vi "Messaging AE.vi"(5 "VI Refnum":refnum<vi>, 7 "Action":T1=enum."Get", 8 "Error In":errorcluster) -> (0 "Error Out":errorcluster, 3 "queue out":refnum<queue>)   [LabVIEW 2019, in "GUI.lvlib"]
doc: "<b>Action</b> Engine\nCreate: Obtains a Queue named after the VI.\nGet: Returns the Queue reference.\nDestroy: Releases the Queue.\n\nUse this VI before and after the main loop. Use the Get action in new APIs."
uses:
  GUI.lvlib
  Controls/Messaging Actions.ctl
  Controls/Messaging Data.ctl
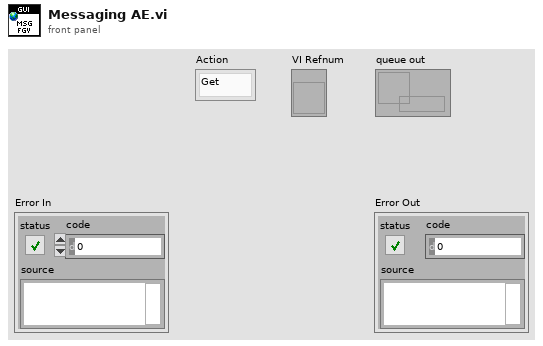
[diagram p1: front panel]
types:
  T1 = typedef "GUI.lvlib/Messaging Actions.ctl" = enum16{"Create", "Get", "Destroy"}
  T2 = typedef "GUI.lvlib/Messaging Data.ctl" = cluster{"Command":string, "Data":variant}
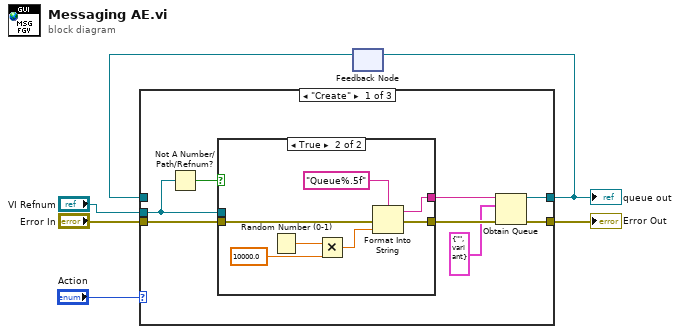
[diagram p0: block diagram]
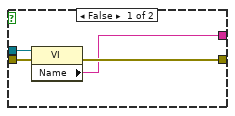
[diagram p2: hidden frame]
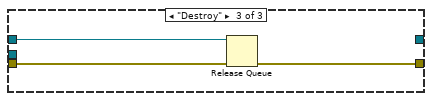
[diagram p4: hidden frame]
diagram:
  n1 = feedback #1() -> (w4:refnum<queue>)  [unwired: 1 in]
  n2 = case shown="\"Create\"" "Action" {
    tunnel: "Error In" -> [w14 w26 w30]
    tunnel: [w7 w26 w29] -> w5
    tunnel: [w12 w27 _] -> w3
    tunnel: w4 -> [_ w27 w28]
    tunnel: "VI Refnum" -> [w11 _ _]
    frame "Create" {
      n3 = Not A Number/Path/Refnum?(number/path/refnum=w11) -> (NaN/Path/Refnum?=w10:bool)
      n4 = case shown="True" w10 {
        tunnel: w14 -> [w18 w25]
        tunnel: [w17 w22] -> w13
        tunnel: w11 -> [w16 _]
        tunnel: [w15 w19] -> w9
        frame False {
          n5 = property class="VI"(reference=w16, error in=w18) -> (error out=w17:errorcluster, "Name"=w15:string)  [unwired: 1 out]
        }
        frame True {
          n6 = Random Number (0-1)() -> (number: 0 to 1=w24:dbl)
          n7 = Multiply(x=w24, y=10000.0) -> (x*y=w21:dbl)
          n8 = Format Into String(format string="Queue%.5f", error in=w25, w21) -> (resulting string=w19:string, error out=w22:errorcluster)  [unwired: 1 in]
        }
      }
      n9 = Obtain Queue(name (unnamed)=w9, element data type=T2 {"Command"="", "Data"=variant} ("Message Data"), error in (no error)=w13) -> (queue out=w12:refnum<queue>, error out=w7:errorcluster)  [unwired: 2 in, 1 out]
    }
    frame "Get", Default {
    }
    frame "Destroy" {
      n10 = Release Queue(queue=w28, error in (no error)=w30) -> (error out=w29:errorcluster)  [unwired: 1 in, 2 out]
    }
  }
  "Error Out" <- w5
  "queue out" <- w3
  n11 = feedback-in #1(w3) -> ()
